vi "Lab Panel V6.00.vi"() -> ()   [LabVIEW 2017] (continued)
                n1128 = Less?(x=w2144, y=2) -> (x < y?=w2142:bool)
                n1129 = local read "DISP LAB01-1"() -> (w2145:T4)
                n1130 = Unbundle By Name(w2145) -> ("STATUS"=w2139:string)
                n1131 = Equal?(x=w2139, y="RUN") -> (x = y?=w2141:bool)
                n1132 = And(x=w2141, y=w2142) -> (x .and. y?=w2140:bool)
                n1133 = case shown="True" w2140 {
                  tunnel: w2145 -> [_ w2150]
                  tunnel: w2144 -> [_ w2154]
                  frame False {
                  }
                  frame True {
                    n1134 = local read "SET LAB01-1"() -> (w2156:T6)
                    n1135 = local read "TDMS LAB01-1"() -> (w2149:refnum<k34>)
                    n1136 = Unbundle(w2156) -> ("CYCLES"=w2147:dbl, "T-RISE mins"=w2153:dbl)  [unwired: 3 out]
                    n1137 = case shown="\"CYCLE TEST\"" w2154 {
                      tunnel: w2153 -> [_ _ w2163]
                      tunnel: [w2158 w2160 w2163] -> w2152
                      tunnel: w2147 -> [w2158 w2160 _]
                      tunnel: ["CHART PASS" "CYCLE PASS" "T-RISE PASS"] -> w2151
                      frame "CHART TEST", Default {
                      }
                      frame "CYCLE TEST" {
                      }
                      frame "T-RISE TEST" {
                      }
                    }
                    n1138 = Unbundle(w2150) -> ("CYCLE"=w2155:dbl)  [unwired: 2 out]
                    n1139 = Increment(x=w2147) -> (x+1=w2148:dbl)
                    n1140 = Greater Or Equal?(x=w2155, y=w2148) -> (x >= y?=w2157:bool)
                    n1141 = case shown="True" w2157 {
                      tunnel: w2152 -> [w2167 _]
                      tunnel: w2151 -> [w2166 _]
                      tunnel: w2150 -> [w2165 _]
                      tunnel: w2149 -> [w2164 _]
                      frame True {
                        n1142 = stacked-sequence {
                          tunnel: w2167 -> [w2171 _]
                          tunnel: w2166 -> [w2169 w2175]
                          tunnel: w2165 -> [_ w2178]
                          tunnel: w2164 -> [w2168 _]
                          frame #0 {
                            n1143 = Build Array(w2169) -> (w2172:string[])
                            n1144 = Build Array(w2171) -> (w2170:dbl[])
                            n1145 = TDMS Write(0:w2168, 5:"TEST PASS", 7:w2172, 9:w2170) -> (15:w2174:errorcluster)  [unwired: 2 in, 3 out]
                            n1146 = local write "data file error"(w2174) -> ()
                          }
                          frame #1 {
                            n1147 = Bundle(cluster=w2178, "STATUS"=w2175) -> (w2176:T4)  [unwired: 2 in]
                            n1148 = local write "RESULT LAB01-1"(TRUE) -> ()
                            n1149 = local write "DISP LAB01-1"(w2176) -> ()
                          }
                        }
                      }
                      frame False {
                      }
                    }
                  }
                }
              }
              frame #1 {
                # "LAB01-2"
                n1150 = Less?(x=w2179, y=2) -> (x < y?=w2182:bool)
                n1151 = local read "DISP LAB01-2"() -> (w2184:T4)
                n1152 = Unbundle(w2184) -> ("STATUS"=w2185:string)  [unwired: 2 out]
                n1153 = Equal?(x=w2185, y="RUN") -> (x = y?=w2181:bool)
                n1154 = And(x=w2181, y=w2182) -> (x .and. y?=w2180:bool)
                n1155 = case shown="True" w2180 {
                  tunnel: w2184 -> [_ w2190]
                  tunnel: w2179 -> [_ w2194]
                  frame False {
                  }
                  frame True {
                    n1156 = local read "SET LAB01-2"() -> (w2196:T5)
                    n1157 = local read "TDMS LAB01-2"() -> (w2189:refnum<k34>)
                    n1158 = Unbundle(w2196) -> ("CYCLES"=w2187:dbl, "T-RISE mins"=w2193:dbl)  [unwired: 3 out]
                    n1159 = case shown="\"T-RISE TEST\"" w2194 {
                      tunnel: w2193 -> [_ _ w2203]
                      tunnel: [w2198 w2200 w2203] -> w2192
                      tunnel: w2187 -> [w2198 w2200 _]
                      tunnel: ["CHART PASS" "CYCLE PASS" "T-RISE PASS"] -> w2191
                      frame "CHART TEST", Default {
                      }
                      frame "CYCLE TEST" {
                      }
                      frame "T-RISE TEST" {
                      }
                    }
                    n1160 = Unbundle(w2190) -> ("CYCLE"=w2195:dbl)  [unwired: 2 out]
                    n1161 = Increment(x=w2187) -> (x+1=w2188:dbl)
                    n1162 = Greater Or Equal?(x=w2195, y=w2188) -> (x >= y?=w2197:bool)
                    n1163 = case shown="True" w2197 {
                      tunnel: w2192 -> [w2207 _]
                      tunnel: w2191 -> [w2206 _]
                      tunnel: w2190 -> [w2205 _]
                      tunnel: w2189 -> [w2204 _]
                      frame True {
                        n1164 = stacked-sequence {
                          tunnel: w2207 -> [w2211 _]
                          tunnel: w2206 -> [w2209 w2215]
                          tunnel: w2205 -> [_ w2218]
                          tunnel: w2204 -> [w2208 _]
                          frame #0 {
                            n1165 = Build Array(w2209) -> (w2212:string[])
                            n1166 = Build Array(w2211) -> (w2210:dbl[])
                            n1167 = TDMS Write(0:w2208, 5:"TEST PASS", 7:w2212, 9:w2210) -> (15:w2214:errorcluster)  [unwired: 2 in, 3 out]
                            n1168 = local write "data file error"(w2214) -> ()
                          }
                          frame #1 {
                            n1169 = Bundle(cluster=w2218, "STATUS"=w2215) -> (w2216:T4)  [unwired: 2 in]
                            n1170 = local write "RESULT LAB01-2"(TRUE) -> ()
                            n1171 = local write "DISP LAB01-2"(w2216) -> ()
                          }
                        }
                      }
                      frame False {
                      }
                    }
                  }
                }
              }
              frame #2 {
                # "LAB02-1"
                n1172 = Less?(x=w2219, y=2) -> (x < y?=w2222:bool)
                n1173 = local read "DISP LAB02-1"() -> (w2224:T4)
                n1174 = Unbundle(w2224) -> ("STATUS"=w2225:string)  [unwired: 2 out]
                n1175 = Equal?(x=w2225, y="RUN") -> (x = y?=w2221:bool)
                n1176 = And(x=w2221, y=w2222) -> (x .and. y?=w2220:bool)
                n1177 = case shown="True" w2220 {
                  tunnel: w2224 -> [_ w2230]
                  tunnel: w2219 -> [_ w2234]
                  frame False {
                  }
                  frame True {
                    n1178 = local read "TDMS LAB02-1"() -> (w2229:refnum<k34>)
                    n1179 = local read "SET LAB02-1"() -> (w2236:T5)
                    n1180 = Unbundle(w2230) -> ("CYCLE"=w2235:dbl)  [unwired: 2 out]
                    n1181 = Unbundle(w2236) -> ("CYCLES"=w2227:dbl, "T-RISE mins"=w2233:dbl)  [unwired: 3 out]
                    n1182 = case shown="\"T-RISE TEST\"" w2234 {
                      tunnel: w2233 -> [_ _ w2243]
                      tunnel: [w2238 w2240 w2243] -> w2232
                      tunnel: w2227 -> [w2238 w2240 _]
                      tunnel: ["CHART PASS" "CYCLE PASS" "T-RISE PASS"] -> w2231
                      frame "CHART TEST", Default {
                      }
                      frame "CYCLE TEST" {
                      }
                      frame "T-RISE TEST" {
                      }
                    }
                    n1183 = Increment(x=w2227) -> (x+1=w2228:dbl)
                    n1184 = Greater Or Equal?(x=w2235, y=w2228) -> (x >= y?=w2237:bool)
                    n1185 = case shown="True" w2237 {
                      tunnel: w2232 -> [w2247 _]
                      tunnel: w2231 -> [w2246 _]
                      tunnel: w2230 -> [w2245 _]
                      tunnel: w2229 -> [w2244 _]
                      frame True {
                        n1186 = stacked-sequence {
                          tunnel: w2247 -> [w2251 _]
                          tunnel: w2246 -> [w2249 w2255]
                          tunnel: w2245 -> [_ w2258]
                          tunnel: w2244 -> [w2248 _]
                          frame #0 {
                            n1187 = Build Array(w2249) -> (w2252:string[])
                            n1188 = Build Array(w2251) -> (w2250:dbl[])
                            n1189 = TDMS Write(0:w2248, 5:"TEST PASS", 7:w2252, 9:w2250) -> (15:w2254:errorcluster)  [unwired: 2 in, 3 out]
                            n1190 = local write "data file error"(w2254) -> ()
                          }
                          frame #1 {
                            n1191 = Bundle(cluster=w2258, "STATUS"=w2255) -> (w2256:T4)  [unwired: 2 in]
                            n1192 = local write "RESULT LAB02-1"(TRUE) -> ()
                            n1193 = local write "DISP LAB02-1"(w2256) -> ()
                          }
                        }
                      }
                      frame False {
                      }
                    }
                  }
                }
              }
              frame #3 {
                # "LAB02-2"
                n1194 = Less?(x=w2259, y=2) -> (x < y?=w2262:bool)
                n1195 = local read "DISP LAB02-2"() -> (w2264:T4)
                n1196 = Unbundle(w2264) -> ("STATUS"=w2265:string)  [unwired: 2 out]
                n1197 = Equal?(x=w2265, y="RUN") -> (x = y?=w2261:bool)
                n1198 = And(x=w2261, y=w2262) -> (x .and. y?=w2260:bool)
                n1199 = case shown="True" w2260 {
                  tunnel: w2264 -> [_ w2270]
                  tunnel: w2259 -> [_ w2274]
                  frame False {
                  }
                  frame True {
                    n1200 = local read "TDMS LAB02-2"() -> (w2269:refnum<k34>)
                    n1201 = local read "SET LAB02-2"() -> (w2276:T5)
                    n1202 = Unbundle(w2270) -> ("CYCLE"=w2275:dbl)  [unwired: 2 out]
                    n1203 = Unbundle(w2276) -> ("CYCLES"=w2267:dbl, "T-RISE mins"=w2273:dbl)  [unwired: 3 out]
                    n1204 = case shown="\"T-RISE TEST\"" w2274 {
                      tunnel: w2273 -> [_ _ w2283]
                      tunnel: [w2278 w2280 w2283] -> w2272
                      tunnel: w2267 -> [w2278 w2280 _]
                      tunnel: ["CHART PASS" "CYCLE PASS" "T-RISE PASS"] -> w2271
                      frame "CHART TEST", Default {
                      }
                      frame "CYCLE TEST" {
                      }
                      frame "T-RISE TEST" {
                      }
                    }
                    n1205 = Increment(x=w2267) -> (x+1=w2268:dbl)
                    n1206 = Greater Or Equal?(x=w2275, y=w2268) -> (x >= y?=w2277:bool)
                    n1207 = case shown="True" w2277 {
                      tunnel: w2272 -> [w2287 _]
                      tunnel: w2271 -> [w2286 _]
                      tunnel: w2270 -> [w2285 _]
                      tunnel: w2269 -> [w2284 _]
                      frame True {
                        n1208 = stacked-sequence {
                          tunnel: w2287 -> [w2291 _]
                          tunnel: w2286 -> [w2289 w2295]
                          tunnel: w2285 -> [_ w2298]
                          tunnel: w2284 -> [w2288 _]
                          frame #0 {
                            n1209 = Build Array(w2289) -> (w2292:string[])
                            n1210 = Build Array(w2291) -> (w2290:dbl[])
                            n1211 = TDMS Write(0:w2288, 5:"TEST PASS", 7:w2292, 9:w2290) -> (15:w2294:errorcluster)  [unwired: 2 in, 3 out]
                            n1212 = local write "data file error"(w2294) -> ()
                          }
                          frame #1 {
                            n1213 = Bundle(cluster=w2298, "STATUS"=w2295) -> (w2296:T4)  [unwired: 2 in]
                            n1214 = local write "RESULT LAB02-2"(TRUE) -> ()
                            n1215 = local write "DISP LAB02-2"(w2296) -> ()
                          }
                        }
                      }
                      frame False {
                      }
                    }
                  }
                }
              }
              frame #4 {
                # "LAB03-1"
                n1216 = Less?(x=w2299, y=2) -> (x < y?=w2302:bool)
                n1217 = local read "DISP LAB03-1"() -> (w2304:T4)
                n1218 = Unbundle(w2304) -> ("STATUS"=w2305:string)  [unwired: 2 out]
                n1219 = Equal?(x=w2305, y="RUN") -> (x = y?=w2301:bool)
                n1220 = And(x=w2301, y=w2302) -> (x .and. y?=w2300:bool)
                n1221 = case shown="True" w2300 {
                  tunnel: w2304 -> [_ w2310]
                  tunnel: w2299 -> [_ w2314]
                  frame False {
                  }
                  frame True {
                    n1222 = local read "TDMS LAB03-1"() -> (w2309:refnum<k34>)
                    n1223 = local read "SET LAB03-1"() -> (w2316:T5)
                    n1224 = Unbundle(w2310) -> ("CYCLE"=w2315:dbl)  [unwired: 2 out]
                    n1225 = Unbundle(w2316) -> ("CYCLES"=w2307:dbl, "T-RISE mins"=w2313:dbl)  [unwired: 3 out]
                    n1226 = case shown="\"T-RISE TEST\"" w2314 {
                      tunnel: w2313 -> [_ _ w2323]
                      tunnel: [w2318 w2320 w2323] -> w2312
                      tunnel: w2307 -> [w2318 w2320 _]
                      tunnel: ["CHART PASS" "CYCLE PASS" "T-RISE PASS"] -> w2311
                      frame "CHART TEST", Default {
                      }
                      frame "CYCLE TEST" {
                      }
                      frame "T-RISE TEST" {
                      }
                    }
                    n1227 = Increment(x=w2307) -> (x+1=w2308:dbl)
                    n1228 = Greater Or Equal?(x=w2315, y=w2308) -> (x >= y?=w2317:bool)
                    n1229 = case shown="True" w2317 {
                      tunnel: w2312 -> [w2327 _]
                      tunnel: w2311 -> [w2326 _]
                      tunnel: w2310 -> [w2325 _]
                      tunnel: w2309 -> [w2324 _]
                      frame True {
                        n1230 = stacked-sequence {
                          tunnel: w2327 -> [w2331 _]
                          tunnel: w2326 -> [w2329 w2335]
                          tunnel: w2325 -> [_ w2338]
                          tunnel: w2324 -> [w2328 _]
                          frame #0 {
                            n1231 = Build Array(w2329) -> (w2332:string[])
                            n1232 = Build Array(w2331) -> (w2330:dbl[])
                            n1233 = TDMS Write(0:w2328, 5:"TEST PASS", 7:w2332, 9:w2330) -> (15:w2334:errorcluster)  [unwired: 2 in, 3 out]
                            n1234 = local write "data file error"(w2334) -> ()
                          }
                          frame #1 {
                            n1235 = Bundle(cluster=w2338, "STATUS"=w2335) -> (w2336:T4)  [unwired: 2 in]
                            n1236 = local write "RESULT LAB03-1"(TRUE) -> ()
                            n1237 = local write "DISP LAB03-1"(w2336) -> ()
                          }
                        }
                      }
                      frame False {
                      }
                    }
                  }
                }
              }
              frame #5 {
                # "LAB03-2"
                n1238 = Less?(x=w2339, y=2) -> (x < y?=w2342:bool)
                n1239 = local read "DISP LAB03-2"() -> (w2344:T4)
                n1240 = Unbundle(w2344) -> ("STATUS"=w2345:string)  [unwired: 2 out]
                n1241 = Equal?(x=w2345, y="RUN") -> (x = y?=w2341:bool)
                n1242 = And(x=w2341, y=w2342) -> (x .and. y?=w2340:bool)
                n1243 = case shown="True" w2340 {
                  tunnel: w2344 -> [_ w2350]
                  tunnel: w2339 -> [_ w2354]
                  frame False {
                  }
                  frame True {
                    n1244 = local read "TDMS LAB03-2"() -> (w2349:refnum<k34>)
                    n1245 = local read "SET LAB03-2"() -> (w2356:T5)
                    n1246 = Unbundle(w2350) -> ("CYCLE"=w2355:dbl)  [unwired: 2 out]
                    n1247 = Unbundle(w2356) -> ("CYCLES"=w2347:dbl, "T-RISE mins"=w2353:dbl)  [unwired: 3 out]
                    n1248 = case shown="\"T-RISE TEST\"" w2354 {
                      tunnel: w2353 -> [_ _ w2363]
                      tunnel: [w2358 w2360 w2363] -> w2352
                      tunnel: w2347 -> [w2358 w2360 _]
                      tunnel: ["CHART PASS" "CYCLE PASS" "T-RISE PASS"] -> w2351
                      frame "CHART TEST", Default {
                      }
                      frame "CYCLE TEST" {
                      }
                      frame "T-RISE TEST" {
                      }
                    }
                    n1249 = Increment(x=w2347) -> (x+1=w2348:dbl)
                    n1250 = Greater Or Equal?(x=w2355, y=w2348) -> (x >= y?=w2357:bool)
                    n1251 = case shown="True" w2357 {
                      tunnel: w2352 -> [w2367 _]
                      tunnel: w2351 -> [w2366 _]
                      tunnel: w2350 -> [w2365 _]
                      tunnel: w2349 -> [w2364 _]
                      frame True {
                        n1252 = stacked-sequence {
                          tunnel: w2367 -> [w2371 _]
                          tunnel: w2366 -> [w2369 w2375]
                          tunnel: w2365 -> [_ w2378]
                          tunnel: w2364 -> [w2368 _]
                          frame #0 {
                            n1253 = Build Array(w2369) -> (w2372:string[])
                            n1254 = Build Array(w2371) -> (w2370:dbl[])
                            n1255 = TDMS Write(0:w2368, 5:"TEST PASS", 7:w2372, 9:w2370) -> (15:w2374:errorcluster)  [unwired: 2 in, 3 out]
                            n1256 = local write "data file error"(w2374) -> ()
                          }
                          frame #1 {
                            n1257 = Bundle(cluster=w2378, "STATUS"=w2375) -> (w2376:T4)  [unwired: 2 in]
                            n1258 = local write "RESULT LAB03-2"(TRUE) -> ()
                            n1259 = local write "DISP LAB03-2"(w2376) -> ()
                          }
                        }
                      }
                      frame False {
                      }
                    }
                  }
                }
              }
              frame #6 {
                # "LAB04-1"
                n1260 = Less?(x=w2379, y=2) -> (x < y?=w2382:bool)
                n1261 = local read "DISP LAB04-1"() -> (w2384:T4)
                n1262 = Unbundle(w2384) -> ("STATUS"=w2385:string)  [unwired: 2 out]
                n1263 = Equal?(x=w2385, y="RUN") -> (x = y?=w2381:bool)
                n1264 = And(x=w2381, y=w2382) -> (x .and. y?=w2380:bool)
                n1265 = case shown="True" w2380 {
                  tunnel: w2384 -> [_ w2390]
                  tunnel: w2379 -> [_ w2394]
                  frame False {
                  }
                  frame True {
                    n1266 = local read "TDMS LAB04-1"() -> (w2389:refnum<k34>)
                    n1267 = local read "SET LAB04-1"() -> (w2396:T5)
                    n1268 = Unbundle(w2390) -> ("CYCLE"=w2395:dbl)  [unwired: 2 out]
                    n1269 = Unbundle(w2396) -> ("CYCLES"=w2387:dbl, "T-RISE mins"=w2393:dbl)  [unwired: 3 out]
                    n1270 = case shown="\"T-RISE TEST\"" w2394 {
                      tunnel: w2393 -> [_ _ w2403]
                      tunnel: [w2398 w2400 w2403] -> w2392
                      tunnel: w2387 -> [w2398 w2400 _]
                      tunnel: ["CHART PASS" "CYCLE PASS" "T-RISE PASS"] -> w2391
                      frame "CHART TEST", Default {
                      }
                      frame "CYCLE TEST" {
                      }
                      frame "T-RISE TEST" {
                      }
                    }
                    n1271 = Increment(x=w2387) -> (x+1=w2388:dbl)
                    n1272 = Greater Or Equal?(x=w2395, y=w2388) -> (x >= y?=w2397:bool)
                    n1273 = case shown="True" w2397 {
                      tunnel: w2392 -> [w2407 _]
                      tunnel: w2391 -> [w2406 _]
                      tunnel: w2390 -> [w2405 _]
                      tunnel: w2389 -> [w2404 _]
                      frame True {
                        n1274 = stacked-sequence {
                          tunnel: w2407 -> [w2411 _]
                          tunnel: w2406 -> [w2409 w2415]
                          tunnel: w2405 -> [_ w2418]
                          tunnel: w2404 -> [w2408 _]
                          frame #0 {
                            n1275 = Build Array(w2409) -> (w2412:string[])
                            n1276 = Build Array(w2411) -> (w2410:dbl[])
                            n1277 = TDMS Write(0:w2408, 5:"TEST PASS", 7:w2412, 9:w2410) -> (15:w2414:errorcluster)  [unwired: 2 in, 3 out]
                            n1278 = local write "data file error"(w2414) -> ()
                          }
                          frame #1 {
                            n1279 = Bundle(cluster=w2418, "STATUS"=w2415) -> (w2416:T4)  [unwired: 2 in]
                            n1280 = local write "RESULT LAB04-1"(TRUE) -> ()
                            n1281 = local write "DISP LAB04-1"(w2416) -> ()
                          }
                        }
                      }
                      frame False {
                      }
                    }
                  }
                }
              }
              frame #7 {
                # "LAB04-2"
                n1282 = Less?(x=w2419, y=2) -> (x < y?=w2422:bool)
                n1283 = local read "DISP LAB04-2"() -> (w2424:T4)
                n1284 = Unbundle(w2424) -> ("STATUS"=w2425:string)  [unwired: 2 out]
                n1285 = Equal?(x=w2425, y="RUN") -> (x = y?=w2421:bool)
                n1286 = And(x=w2421, y=w2422) -> (x .and. y?=w2420:bool)
                n1287 = case shown="True" w2420 {
                  tunnel: w2424 -> [_ w2430]
                  tunnel: w2419 -> [_ w2434]
                  frame False {
                  }
                  frame True {
                    n1288 = local read "TDMS LAB04-2"() -> (w2429:refnum<k34>)
                    n1289 = local read "SET LAB04-2"() -> (w2436:T5)
                    n1290 = Unbundle(w2430) -> ("CYCLE"=w2435:dbl)  [unwired: 2 out]
                    n1291 = Unbundle(w2436) -> ("CYCLES"=w2427:dbl, "T-RISE mins"=w2433:dbl)  [unwired: 3 out]
                    n1292 = case shown="\"T-RISE TEST\"" w2434 {
                      tunnel: w2433 -> [_ _ w2443]
                      tunnel: [w2438 w2440 w2443] -> w2432
                      tunnel: w2427 -> [w2438 w2440 _]
                      tunnel: ["CHART PASS" "CYCLE PASS" "T-RISE PASS"] -> w2431
                      frame "CHART TEST", Default {
                      }
                      frame "CYCLE TEST" {
                      }
                      frame "T-RISE TEST" {
                      }
                    }
                    n1293 = Increment(x=w2427) -> (x+1=w2428:dbl)
                    n1294 = Greater Or Equal?(x=w2435, y=w2428) -> (x >= y?=w2437:bool)
                    n1295 = case shown="True" w2437 {
                      tunnel: w2432 -> [w2447 _]
                      tunnel: w2431 -> [w2446 _]
                      tunnel: w2430 -> [w2445 _]
                      tunnel: w2429 -> [w2444 _]
                      frame True {
                        n1296 = stacked-sequence {
                          tunnel: w2447 -> [w2451 _]
                          tunnel: w2446 -> [w2449 w2455]
                          tunnel: w2445 -> [_ w2458]
                          tunnel: w2444 -> [w2448 _]
                          frame #0 {
                            n1297 = Build Array(w2449) -> (w2452:string[])
                            n1298 = Build Array(w2451) -> (w2450:dbl[])
                            n1299 = TDMS Write(0:w2448, 5:"TEST PASS", 7:w2452, 9:w2450) -> (15:w2454:errorcluster)  [unwired: 2 in, 3 out]
                            n1300 = local write "data file error"(w2454) -> ()
                          }
                          frame #1 {
                            n1301 = Bundle(cluster=w2458, "STATUS"=w2455) -> (w2456:T4)  [unwired: 2 in]
                            n1302 = local write "RESULT LAB04-2"(TRUE) -> ()
                            n1303 = local write "DISP LAB04-2"(w2456) -> ()
                          }
                        }
                      }
                      frame False {
                      }
                    }
                  }
                }
              }
              frame #8 {
                # "LAB05-1"
                n1304 = Less?(x=w2459, y=2) -> (x < y?=w2462:bool)
                n1305 = local read "DISP LAB05-1"() -> (w2464:T4)
                n1306 = Unbundle(w2464) -> ("STATUS"=w2465:string)  [unwired: 2 out]
                n1307 = Equal?(x=w2465, y="RUN") -> (x = y?=w2461:bool)
                n1308 = And(x=w2461, y=w2462) -> (x .and. y?=w2460:bool)
                n1309 = case shown="True" w2460 {
                  tunnel: w2464 -> [_ w2470]
                  tunnel: w2459 -> [_ w2474]
                  frame False {
                  }
                  frame True {
                    n1310 = local read "TDMS LAB05-1"() -> (w2469:refnum<k34>)
                    n1311 = local read "SET LAB05-1"() -> (w2476:T5)
                    n1312 = Unbundle(w2470) -> ("CYCLE"=w2475:dbl)  [unwired: 2 out]
                    n1313 = Unbundle(w2476) -> ("CYCLES"=w2467:dbl, "T-RISE mins"=w2473:dbl)  [unwired: 3 out]
                    n1314 = case shown="\"T-RISE TEST\"" w2474 {
                      tunnel: w2473 -> [_ _ w2483]
                      tunnel: [w2478 w2480 w2483] -> w2472
                      tunnel: w2467 -> [w2478 w2480 _]
                      tunnel: ["CHART PASS" "CYCLE PASS" "T-RISE PASS"] -> w2471
                      frame "CHART TEST", Default {
                      }
                      frame "CYCLE TEST" {
                      }
                      frame "T-RISE TEST" {
                      }
                    }
                    n1315 = Increment(x=w2467) -> (x+1=w2468:dbl)
                    n1316 = Greater Or Equal?(x=w2475, y=w2468) -> (x >= y?=w2477:bool)
                    n1317 = case shown="True" w2477 {
                      tunnel: w2472 -> [w2487 _]
                      tunnel: w2471 -> [w2486 _]
                      tunnel: w2470 -> [w2485 _]
                      tunnel: w2469 -> [w2484 _]
                      frame True {
                        n1318 = stacked-sequence {
                          tunnel: w2487 -> [w2491 _]
                          tunnel: w2486 -> [w2489 w2495]
                          tunnel: w2485 -> [_ w2498]
                          tunnel: w2484 -> [w2488 _]
                          frame #0 {
                            n1319 = Build Array(w2489) -> (w2492:string[])
                            n1320 = Build Array(w2491) -> (w2490:dbl[])
                            n1321 = TDMS Write(0:w2488, 5:"TEST PASS", 7:w2492, 9:w2490) -> (15:w2494:errorcluster)  [unwired: 2 in, 3 out]
                            n1322 = local write "data file error"(w2494) -> ()
                          }
                          frame #1 {
                            n1323 = Bundle(cluster=w2498, "STATUS"=w2495) -> (w2496:T4)  [unwired: 2 in]
                            n1324 = local write "RESULT LAB05-1"(TRUE) -> ()
                            n1325 = local write "DISP LAB05-1"(w2496) -> ()
                          }
                        }
                      }
                      frame False {
                      }
                    }
                  }
                }
              }
              frame #9 {
                # "LAB05-2"
                n1326 = Less?(x=w2499, y=2) -> (x < y?=w2502:bool)
                n1327 = local read "DISP LAB05-2"() -> (w2504:T4)
                n1328 = Unbundle(w2504) -> ("STATUS"=w2505:string)  [unwired: 2 out]
                n1329 = Equal?(x=w2505, y="RUN") -> (x = y?=w2501:bool)
                n1330 = And(x=w2501, y=w2502) -> (x .and. y?=w2500:bool)
                n1331 = case shown="True" w2500 {
                  tunnel: w2504 -> [_ w2510]
                  tunnel: w2499 -> [_ w2514]
                  frame False {
                  }
                  frame True {
                    n1332 = local read "TDMS LAB05-2"() -> (w2509:refnum<k34>)
                    n1333 = local read "SET LAB05-2"() -> (w2516:T5)
                    n1334 = Unbundle(w2510) -> ("CYCLE"=w2515:dbl)  [unwired: 2 out]
                    n1335 = Unbundle(w2516) -> ("CYCLES"=w2507:dbl, "T-RISE mins"=w2513:dbl)  [unwired: 3 out]
                    n1336 = case shown="\"T-RISE TEST\"" w2514 {
                      tunnel: w2513 -> [_ _ w2523]
                      tunnel: [w2518 w2520 w2523] -> w2512
                      tunnel: w2507 -> [w2518 w2520 _]
                      tunnel: ["CHART PASS" "CYCLE PASS" "T-RISE PASS"] -> w2511
                      frame "CHART TEST", Default {
                      }
                      frame "CYCLE TEST" {
                      }
                      frame "T-RISE TEST" {
                      }
                    }
                    n1337 = Increment(x=w2507) -> (x+1=w2508:dbl)
                    n1338 = Greater Or Equal?(x=w2515, y=w2508) -> (x >= y?=w2517:bool)
                    n1339 = case shown="True" w2517 {
                      tunnel: w2512 -> [w2527 _]
                      tunnel: w2511 -> [w2526 _]
                      tunnel: w2510 -> [w2525 _]
                      tunnel: w2509 -> [w2524 _]
                      frame True {
                        n1340 = stacked-sequence {
                          tunnel: w2527 -> [w2531 _]
                          tunnel: w2526 -> [w2529 w2535]
                          tunnel: w2525 -> [_ w2538]
                          tunnel: w2524 -> [w2528 _]
                          frame #0 {
                            n1341 = Build Array(w2529) -> (w2532:string[])
                            n1342 = Build Array(w2531) -> (w2530:dbl[])
                            n1343 = TDMS Write(0:w2528, 5:"TEST PASS", 7:w2532, 9:w2530) -> (15:w2534:errorcluster)  [unwired: 2 in, 3 out]
                            n1344 = local write "data file error"(w2534) -> ()
                          }
                          frame #1 {
                            n1345 = Bundle(cluster=w2538, "STATUS"=w2535) -> (w2536:T4)  [unwired: 2 in]
                            n1346 = local write "RESULT LAB05-2"(TRUE) -> ()
                            n1347 = local write "DISP LAB05-2"(w2536) -> ()
                          }
                        }
                      }
                      frame False {
                      }
                    }
                  }
                }
              }
            }
          }
          frame #6 {
            # "check if test cycles reached for temperature rise test"
            n1348 = stacked-sequence {
              tunnel: w2568 -> [_ _ _ _ _ _ _ _ _ _]
              tunnel: w2567 -> [_ _ _ _ _ _ _ _ _ _]
              tunnel: w2566 -> [_ _ _ _ _ _ _ _ _ _]
              tunnel: w2565 -> [_ _ _ _ _ _ _ _ _ _]
              tunnel: w2564 -> [_ _ _ _ _ _ _ _ _ _]
              tunnel: w2563 -> [_ _ _ _ _ _ _ _ _ _]
              tunnel: w2562 -> [_ _ _ _ _ _ _ _ _ _]
              tunnel: w2561 -> [_ _ _ _ _ _ _ _ _ _]
              tunnel: w2560 -> [_ _ _ _ _ _ _ _ _ _]
              tunnel: w2559 -> [_ _ _ _ _ _ _ _ _ _]
              tunnel: w2558 -> [w2574 _ _ _ _ _ _ _ _ _]
              tunnel: w2548 -> [w2569 _ _ _ _ _ _ _ _ _]
              tunnel: w2557 -> [_ w2600 _ _ _ _ _ _ _ _]
              tunnel: w2556 -> [_ _ w2630 _ _ _ _ _ _ _]
              tunnel: w2555 -> [_ _ _ w2660 _ _ _ _ _ _]
              tunnel: w2554 -> [_ _ _ _ w2690 _ _ _ _ _]
              tunnel: w2553 -> [_ _ _ _ _ w2720 _ _ _ _]
              tunnel: w2552 -> [_ _ _ _ _ _ w2750 _ _ _]
              tunnel: w2551 -> [_ _ _ _ _ _ _ w2780 _ _]
              tunnel: w2550 -> [_ _ _ _ _ _ _ _ w2810 _]
              tunnel: w2549 -> [_ _ _ _ _ _ _ _ _ w2840]
              tunnel: w2547 -> [_ w2599 _ _ _ _ _ _ _ _]
              tunnel: w2546 -> [_ _ w2629 _ _ _ _ _ _ _]
              tunnel: w2545 -> [_ _ _ w2659 _ _ _ _ _ _]
              tunnel: w2544 -> [_ _ _ _ w2689 _ _ _ _ _]
              tunnel: w2543 -> [_ _ _ _ _ w2719 _ _ _ _]
              tunnel: w2542 -> [_ _ _ _ _ _ w2749 _ _ _]
              tunnel: w2541 -> [_ _ _ _ _ _ _ w2779 _ _]
              tunnel: w2540 -> [_ _ _ _ _ _ _ _ w2809 _]
              tunnel: w2539 -> [_ _ _ _ _ _ _ _ _ w2839]
              frame #0 {
                # "LAB01-1"
                n1349 = Equal?(x=w2574, y=2) -> (x = y?=w2572:bool)
                n1350 = local read "DISP LAB01-1"() -> (w2575:T4)
                n1351 = Unbundle By Name(w2575) -> ("STATUS"=w2576:string)
                n1352 = Equal?(x=w2576, y="RUN") -> (x = y?=w2571:bool)
                n1353 = And(x=w2571, y=w2572) -> (x .and. y?=w2570:bool)
                n1354 = case shown="True" w2570 {
                  tunnel: w2575 -> [_ w2579]
                  tunnel: w2569 -> [_ w2582]
                  frame False {
                  }
                  frame True {
                    n1355 = Unbundle By Name(w2579) -> ("CYCLE"=w2583:dbl)
                    n1356 = local read "SET LAB01-1"() -> (w2581:T6)
                    n1357 = local read "TDMS LAB01-1"() -> (w2578:refnum<k34>)
                    n1358 = Unbundle(w2581) -> ("T-RISE mins"=w2580:dbl)  [unwired: 4 out]
                    n1359 = Greater Or Equal?(x=w2583, y=w2582) -> (x >= y?=w2584:bool)
                    n1360 = case shown="True" w2584 {
                      tunnel: w2580 -> [w2587 _]
                      tunnel: w2579 -> [w2586 _]
                      tunnel: w2578 -> [w2585 _]
                      frame True {
                        n1361 = stacked-sequence {
                          tunnel: w2587 -> [w2590 _]
                          tunnel: w2586 -> [_ w2595]
                          tunnel: w2585 -> [w2588 _]
                          frame #0 {
                            n1362 = Build Array("T-RISE") -> (w2592:string[])
                            n1363 = Build Array(w2590) -> (w2591:dbl[])
                            n1364 = TDMS Write(0:w2588, 5:"TEST PASS", 7:w2592, 9:w2591) -> (15:w2594:errorcluster)  [unwired: 2 in, 3 out]
                            n1365 = local write "data file error"(w2594) -> ()
                          }
                          frame #1 {
                            n1366 = Bundle(cluster=w2595, "STATUS"="T-RISE PASS") -> (w2597:T4)  [unwired: 2 in]
                            n1367 = local write "RESULT LAB01-1"(TRUE) -> ()
                            n1368 = local write "DISP LAB01-1"(w2597) -> ()
                          }
                        }
                      }
                      frame False {
                      }
                    }
                  }
                }
              }
              frame #1 {
                # "LAB01-2"
                n1369 = Equal?(x=w2600, y=2) -> (x = y?=w2603:bool)
                n1370 = local read "DISP LAB01-2"() -> (w2605:T4)
                n1371 = Unbundle(w2605) -> ("STATUS"=w2606:string)  [unwired: 2 out]
                n1372 = Equal?(x=w2606, y="RUN") -> (x = y?=w2602:bool)
                n1373 = And(x=w2602, y=w2603) -> (x .and. y?=w2601:bool)
                n1374 = case shown="True" w2601 {
                  tunnel: w2605 -> [_ w2609]
                  tunnel: w2599 -> [_ w2612]
                  frame False {
                  }
                  frame True {
                    n1375 = local read "SET LAB01-2"() -> (w2611:T5)
                    n1376 = local read "TDMS LAB01-2"() -> (w2608:refnum<k34>)
                    n1377 = Unbundle(w2609) -> ("CYCLE"=w2613:dbl)  [unwired: 2 out]
                    n1378 = Unbundle(w2611) -> ("T-RISE mins"=w2610:dbl)  [unwired: 4 out]
                    n1379 = Greater Or Equal?(x=w2613, y=w2612) -> (x >= y?=w2614:bool)
                    n1380 = case shown="True" w2614 {
                      tunnel: w2610 -> [w2617 _]
                      tunnel: w2609 -> [w2616 _]
                      tunnel: w2608 -> [w2615 _]
                      frame True {
                        n1381 = stacked-sequence {
                          tunnel: w2617 -> [w2620 _]
                          tunnel: w2616 -> [_ w2625]
                          tunnel: w2615 -> [w2618 _]
                          frame #0 {
                            n1382 = Build Array("T-RISE") -> (w2622:string[])
                            n1383 = Build Array(w2620) -> (w2621:dbl[])
                            n1384 = TDMS Write(0:w2618, 5:"TEST PASS", 7:w2622, 9:w2621) -> (15:w2624:errorcluster)  [unwired: 2 in, 3 out]
                            n1385 = local write "data file error"(w2624) -> ()
                          }
                          frame #1 {
                            n1386 = Bundle(cluster=w2625, "STATUS"="T-RISE PASS") -> (w2627:T4)  [unwired: 2 in]
                            n1387 = local write "RESULT LAB01-2"(TRUE) -> ()
                            n1388 = local write "DISP LAB01-2"(w2627) -> ()
                          }
                        }
                      }
                      frame False {
                      }
                    }
                  }
                }
              }
              frame #2 {
                # "LAB02-1"
                n1389 = Equal?(x=w2630, y=2) -> (x = y?=w2633:bool)
                n1390 = local read "DISP LAB02-1"() -> (w2635:T4)
                n1391 = Unbundle(w2635) -> ("STATUS"=w2636:string)  [unwired: 2 out]
                n1392 = Equal?(x=w2636, y="RUN") -> (x = y?=w2632:bool)
                n1393 = And(x=w2632, y=w2633) -> (x .and. y?=w2631:bool)
                n1394 = case shown="True" w2631 {
                  tunnel: w2635 -> [_ w2639]
                  tunnel: w2629 -> [_ w2642]
                  frame False {
                  }
                  frame True {
                    n1395 = local read "SET LAB02-1"() -> (w2641:T5)
                    n1396 = local read "TDMS LAB02-1"() -> (w2638:refnum<k34>)
                    n1397 = Unbundle(w2639) -> ("CYCLE"=w2643:dbl)  [unwired: 2 out]
                    n1398 = Unbundle(w2641) -> ("T-RISE mins"=w2640:dbl)  [unwired: 4 out]
                    n1399 = Greater Or Equal?(x=w2643, y=w2642) -> (x >= y?=w2644:bool)
                    n1400 = case shown="True" w2644 {
                      tunnel: w2640 -> [w2647 _]
                      tunnel: w2639 -> [w2646 _]
                      tunnel: w2638 -> [w2645 _]
                      frame True {
                        n1401 = stacked-sequence {
                          tunnel: w2647 -> [w2650 _]
                          tunnel: w2646 -> [_ w2655]
                          tunnel: w2645 -> [w2648 _]
                          frame #0 {
                            n1402 = Build Array("T-RISE") -> (w2652:string[])
                            n1403 = Build Array(w2650) -> (w2651:dbl[])
                            n1404 = TDMS Write(0:w2648, 5:"TEST PASS", 7:w2652, 9:w2651) -> (15:w2654:errorcluster)  [unwired: 2 in, 3 out]
                            n1405 = local write "data file error"(w2654) -> ()
                          }
                          frame #1 {
                            n1406 = Bundle(cluster=w2655, "STATUS"="T-RISE PASS") -> (w2657:T4)  [unwired: 2 in]
                            n1407 = local write "RESULT LAB02-1"(TRUE) -> ()
                            n1408 = local write "DISP LAB02-1"(w2657) -> ()
                          }
                        }
                      }
                      frame False {
                      }
                    }
                  }
                }
              }
              frame #3 {
                # "LAB02-2"
                n1409 = Equal?(x=w2660, y=2) -> (x = y?=w2663:bool)
                n1410 = local read "DISP LAB02-2"() -> (w2665:T4)
                n1411 = Unbundle(w2665) -> ("STATUS"=w2666:string)  [unwired: 2 out]
                n1412 = Equal?(x=w2666, y="RUN") -> (x = y?=w2662:bool)
                n1413 = And(x=w2662, y=w2663) -> (x .and. y?=w2661:bool)
                n1414 = case shown="True" w2661 {
                  tunnel: w2665 -> [_ w2669]
                  tunnel: w2659 -> [_ w2672]
                  frame False {
                  }
                  frame True {
                    n1415 = local read "SET LAB02-2"() -> (w2671:T5)
                    n1416 = local read "TDMS LAB02-2"() -> (w2668:refnum<k34>)
                    n1417 = Unbundle(w2669) -> ("CYCLE"=w2673:dbl)  [unwired: 2 out]
                    n1418 = Unbundle(w2671) -> ("T-RISE mins"=w2670:dbl)  [unwired: 4 out]
                    n1419 = Greater Or Equal?(x=w2673, y=w2672) -> (x >= y?=w2674:bool)
                    n1420 = case shown="True" w2674 {
                      tunnel: w2670 -> [w2677 _]
                      tunnel: w2669 -> [w2676 _]
                      tunnel: w2668 -> [w2675 _]
                      frame True {
                        n1421 = stacked-sequence {
                          tunnel: w2677 -> [w2680 _]
                          tunnel: w2676 -> [_ w2685]
                          tunnel: w2675 -> [w2678 _]
                          frame #0 {
                            n1422 = Build Array("T-RISE") -> (w2682:string[])
                            n1423 = Build Array(w2680) -> (w2681:dbl[])
                            n1424 = TDMS Write(0:w2678, 5:"TEST PASS", 7:w2682, 9:w2681) -> (15:w2684:errorcluster)  [unwired: 2 in, 3 out]
                            n1425 = local write "data file error"(w2684) -> ()
                          }
                          frame #1 {
                            n1426 = Bundle(cluster=w2685, "STATUS"="T-RISE PASS") -> (w2687:T4)  [unwired: 2 in]
                            n1427 = local write "RESULT LAB02-2"(TRUE) -> ()
                            n1428 = local write "DISP LAB02-2"(w2687) -> ()
                          }
                        }
                      }
                      frame False {
                      }
                    }
                  }
                }
              }
              frame #4 {
                # "LAB03-1"
                n1429 = Equal?(x=w2690, y=2) -> (x = y?=w2693:bool)
                n1430 = local read "DISP LAB03-1"() -> (w2695:T4)
                n1431 = Unbundle(w2695) -> ("STATUS"=w2696:string)  [unwired: 2 out]
                n1432 = Equal?(x=w2696, y="RUN") -> (x = y?=w2692:bool)
                n1433 = And(x=w2692, y=w2693) -> (x .and. y?=w2691:bool)
                n1434 = case shown="True" w2691 {
                  tunnel: w2695 -> [_ w2699]
                  tunnel: w2689 -> [_ w2702]
                  frame False {
                  }
                  frame True {
                    n1435 = local read "SET LAB03-1"() -> (w2701:T5)
                    n1436 = local read "TDMS LAB03-1"() -> (w2698:refnum<k34>)
                    n1437 = Unbundle(w2699) -> ("CYCLE"=w2703:dbl)  [unwired: 2 out]
                    n1438 = Unbundle(w2701) -> ("T-RISE mins"=w2700:dbl)  [unwired: 4 out]
                    n1439 = Greater Or Equal?(x=w2703, y=w2702) -> (x >= y?=w2704:bool)
                    n1440 = case shown="True" w2704 {
                      tunnel: w2700 -> [w2707 _]
                      tunnel: w2699 -> [w2706 _]
                      tunnel: w2698 -> [w2705 _]
                      frame True {
                        n1441 = stacked-sequence {
                          tunnel: w2707 -> [w2710 _]
                          tunnel: w2706 -> [_ w2715]
                          tunnel: w2705 -> [w2708 _]
                          frame #0 {
                            n1442 = Build Array("T-RISE") -> (w2712:string[])
                            n1443 = Build Array(w2710) -> (w2711:dbl[])
                            n1444 = TDMS Write(0:w2708, 5:"TEST PASS", 7:w2712, 9:w2711) -> (15:w2714:errorcluster)  [unwired: 2 in, 3 out]
                            n1445 = local write "data file error"(w2714) -> ()
                          }
                          frame #1 {
                            n1446 = Bundle(cluster=w2715, "STATUS"="T-RISE PASS") -> (w2717:T4)  [unwired: 2 in]
                            n1447 = local write "RESULT LAB03-1"(TRUE) -> ()
                            n1448 = local write "DISP LAB03-1"(w2717) -> ()
                          }
                        }
                      }
                      frame False {
                      }
                    }
                  }
                }
              }
              frame #5 {
                # "LAB03-2"
                n1449 = Equal?(x=w2720, y=2) -> (x = y?=w2723:bool)
                n1450 = local read "DISP LAB03-2"() -> (w2725:T4)
                n1451 = Unbundle(w2725) -> ("STATUS"=w2726:string)  [unwired: 2 out]
                n1452 = Equal?(x=w2726, y="RUN") -> (x = y?=w2722:bool)
                n1453 = And(x=w2722, y=w2723) -> (x .and. y?=w2721:bool)
                n1454 = case shown="True" w2721 {
                  tunnel: w2725 -> [_ w2729]
                  tunnel: w2719 -> [_ w2732]
                  frame False {
                  }
                  frame True {
                    n1455 = local read "SET LAB03-2"() -> (w2731:T5)
                    n1456 = local read "TDMS LAB03-2"() -> (w2728:refnum<k34>)
                    n1457 = Unbundle(w2729) -> ("CYCLE"=w2733:dbl)  [unwired: 2 out]
                    n1458 = Unbundle(w2731) -> ("T-RISE mins"=w2730:dbl)  [unwired: 4 out]
                    n1459 = Greater Or Equal?(x=w2733, y=w2732) -> (x >= y?=w2734:bool)
                    n1460 = case shown="True" w2734 {
                      tunnel: w2730 -> [w2737 _]
                      tunnel: w2729 -> [w2736 _]
                      tunnel: w2728 -> [w2735 _]
                      frame True {
                        n1461 = stacked-sequence {
                          tunnel: w2737 -> [w2740 _]
                          tunnel: w2736 -> [_ w2745]
                          tunnel: w2735 -> [w2738 _]
                          frame #0 {
                            n1462 = Build Array("T-RISE") -> (w2742:string[])
                            n1463 = Build Array(w2740) -> (w2741:dbl[])
                            n1464 = TDMS Write(0:w2738, 5:"TEST PASS", 7:w2742, 9:w2741) -> (15:w2744:errorcluster)  [unwired: 2 in, 3 out]
                            n1465 = local write "data file error"(w2744) -> ()
                          }
                          frame #1 {
                            n1466 = Bundle(cluster=w2745, "STATUS"="T-RISE PASS") -> (w2747:T4)  [unwired: 2 in]
                            n1467 = local write "RESULT LAB03-2"(TRUE) -> ()
                            n1468 = local write "DISP LAB03-2"(w2747) -> ()
                          }
                        }
                      }
                      frame False {
                      }
                    }
                  }
                }
              }
              frame #6 {
                # "LAB04-1"
                n1469 = Equal?(x=w2750, y=2) -> (x = y?=w2753:bool)
                n1470 = local read "DISP LAB04-1"() -> (w2755:T4)
                n1471 = Unbundle(w2755) -> ("STATUS"=w2756:string)  [unwired: 2 out]
                n1472 = Equal?(x=w2756, y="RUN") -> (x = y?=w2752:bool)
                n1473 = And(x=w2752, y=w2753) -> (x .and. y?=w2751:bool)
                n1474 = case shown="True" w2751 {
                  tunnel: w2755 -> [_ w2759]
                  tunnel: w2749 -> [_ w2762]
                  frame False {
                  }
                  frame True {
                    n1475 = local read "SET LAB04-1"() -> (w2761:T5)
                    n1476 = local read "TDMS LAB04-1"() -> (w2758:refnum<k34>)
                    n1477 = Unbundle(w2759) -> ("CYCLE"=w2763:dbl)  [unwired: 2 out]
                    n1478 = Unbundle(w2761) -> ("T-RISE mins"=w2760:dbl)  [unwired: 4 out]
                    n1479 = Greater Or Equal?(x=w2763, y=w2762) -> (x >= y?=w2764:bool)
                    n1480 = case shown="True" w2764 {
                      tunnel: w2760 -> [w2767 _]
                      tunnel: w2759 -> [w2766 _]
                      tunnel: w2758 -> [w2765 _]
                      frame True {
                        n1481 = stacked-sequence {
                          tunnel: w2767 -> [w2770 _]
                          tunnel: w2766 -> [_ w2775]
                          tunnel: w2765 -> [w2768 _]
                          frame #0 {
                            n1482 = Build Array("T-RISE") -> (w2772:string[])
                            n1483 = Build Array(w2770) -> (w2771:dbl[])
                            n1484 = TDMS Write(0:w2768, 5:"TEST PASS", 7:w2772, 9:w2771) -> (15:w2774:errorcluster)  [unwired: 2 in, 3 out]
                            n1485 = local write "data file error"(w2774) -> ()
